vi "SelectHandle.vi"(8 "error in (no error)":errorcluster, 11 "ClassIn":refnum<class "Keysight335XX.lvclass">) -> (0 "error out":errorcluster, 3 "ClassOut":refnum<class "Keysight335XX.lvclass">)   [LabVIEW 2014, in "FGenPlugins.lvlib" / "Keysight335XX.lvclass"]
uses:
  Keysight335XX.lvclass
  <vilib>/Utility/error.llb/Error Cluster From Error Code.vi
  <vilib>/ErrorRing/Error Ring.xnode
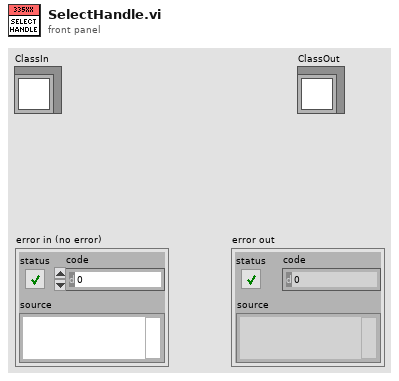
[diagram p1: front panel]
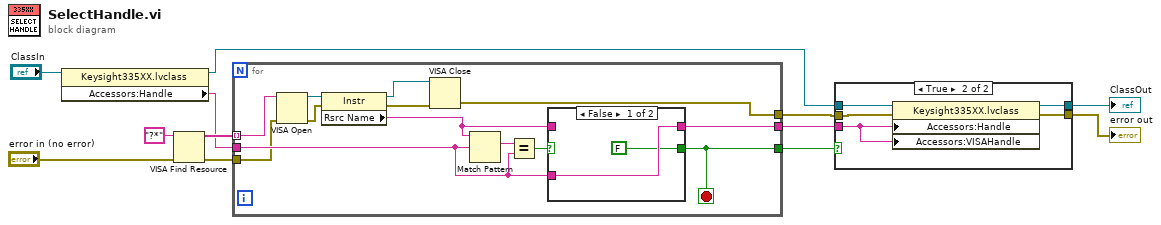
[diagram p0: block diagram]
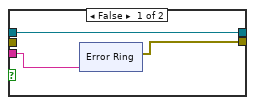
[diagram p2: hidden frame]
diagram:
  n1 = property class="Keysight335XX.lvclass"(reference="ClassIn") -> (reference out=w3:refnum<class "Keysight335XX.lvclass">, "Accessors:Handle"=w8:string)  [unwired: 1 in, 1 out]
  n2 = VISA Find Resource(8:"error in (no error)", 11:"?*" ("expression (\"?*\")")) -> (0:w5:errorcluster, 3:w9:string[])  [unwired: 1 in, 1 out]
  n3 = for {
    tunnel: w9 -> [w21] mode=indexing
    tunnel: w8 -> [w22]
    tunnel: [w23] -> w2
    tunnel: w5 -> [w17]
    tunnel: [w14] -> w1
    tunnel: [w13] -> w4
    stop <- w13 stop-if-true
    n4 = VISA Open(error in (no error)=w17, VISA resource name=w21) -> (VISA resource name=w20:refnum<visa-resource-name>, error out=w16:errorcluster)  [unwired: 3 in]
    n5 = property class="Instr"(reference=w20, error in=w16) -> (reference out=w18:refnum<visa-resource-name>, error out=w15:errorcluster, "Rsrc Name"=w19:string)
    n6 = VISA Close(VISA resource name=w18, error in (no error)=w15) -> (error out=w14:errorcluster)
    n7 = Match Pattern(string=w19, regular expression=w22) -> (match substring=w25:string)  [unwired: 1 in, 3 out]
    n8 = Equal?(x=w25, y=w22) -> (x = y?=w24:bool)
    n9 = case shown="False" w24 {
      selector: w24 -> [_ w28]
      tunnel: w19 -> [_ w29]
      tunnel: [w27 w29] -> w23
      tunnel: w22 -> [w27 _]
      tunnel: [FALSE w28] -> w13
      frame False {
      }
      frame True {
      }
    }
  }
  n10 = case shown="True" w4 {
    tunnel: [w32 w44] -> w7
    tunnel: [w30 w43] -> w6
    tunnel: w3 -> [w32 w42]
    tunnel: w2 -> [w31 w41]
    tunnel: w1 -> [_ w40]
    frame False {
      n11 = xnode "Error Ring"("parameter 0"=w31) -> ("error out"=w30:errorcluster)
    }
    frame True {
      n12 = property class="Keysight335XX.lvclass"(reference=w42, error in=w40, "Accessors:Handle"=w41, "Accessors:VISAHandle"=w41) -> (reference out=w44:refnum<class "Keysight335XX.lvclass">, error out=w43:errorcluster)
    }
  }
  "error out" <- w6
  "ClassOut" <- w7
